vi "Discard One Character.vi"(1 "String":string) -> (0 "Remaining String":string)   [LabVIEW 2016]
doc: "This simple VI returns a string with the first character removed."
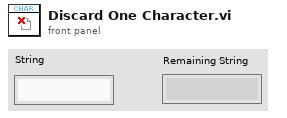
[diagram p1: front panel]
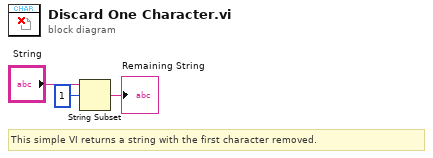
[diagram p0: block diagram]
diagram:
  # "This simple VI returns a string with the first character removed."
  n1 = String Subset(string="String", offset (0)=1) -> (substring=→"Remaining String":string)  [unwired: 1 in]
